vi "Threshold Value Settings.vi"() -> (1 "Threshold Value Settings 2":T1={"Start at"=0.0, "Increment of"=5.0, "Stop at"=15.0, "No. of iterations"=10.0, "Assumed Time Delay"=800.0, "Th high"=90.0, "Verification RT"=1000.0, "Settling Time"=10, "Name of Output"="GFP", "Th Low"=90.0})   [LabVIEW 2014]
doc: "This VI is used to set the initial properties for performing threshold value analysis."
uses:
  Threshold Set.ctl
panel:
  in  "stop":bool
  in  "Threshold Value Settings":T1={"Start at"=0.0, "Increment of"=5.0, "Stop at"=20.0, "No. of iterations"=5.0, "Assumed Time Delay"=1500.0, "Th high"=90.0, "Verification RT"=1500.0, "Settling Time"=500, "Name of Output"="GFP", "Th Low"=40.0}
  # "Input concentration values"
  # "% Acceptance of consistency"
  # "Input concentration values"
  # "% Acceptance of consistency"
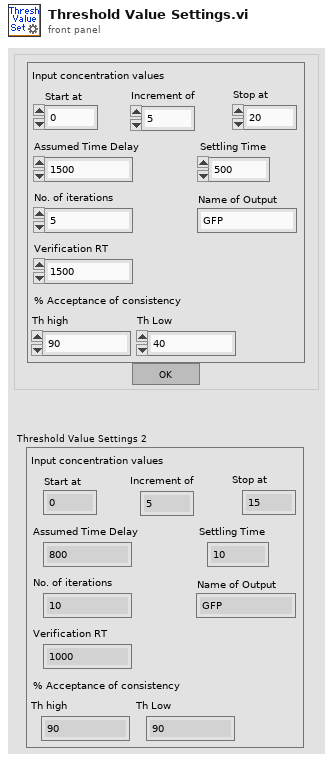
[diagram p1: front panel]
types:
  T1 = typedef "Threshold Set.ctl" = cluster{"Start at":dbl, "Increment of":dbl, "Stop at":dbl, "No. of iterations":dbl, "Assumed Time Delay":dbl, "Th high":dbl, "Verification RT":dbl, "Settling Time":i32, "Name of Output":string, "Th Low":dbl}
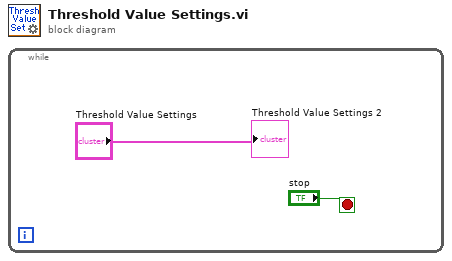
[diagram p0: block diagram]
diagram:
  n1 = while {
    stop <- "stop" stop-if-true
    "Threshold Value Settings 2" <- "Threshold Value Settings"
  }
